vi "Find Exchanges.vi"(8 "error in (no error)":errorcluster caption="entrée d'erreur (pas d'erreur)", 10 "Position":i32, 11 "Exchanges en entrée":refnum<class "Exchanges.lvclass"> caption="DNL_LabVIEW Object in") -> (0 "error out":errorcluster caption="sortie d'erreur", 1 "Parameters":T1, 2 "found?":bool, 3 "Exchanges en sortie":refnum<class "Exchanges.lvclass"> caption="DNL_LabVIEW Object out")   [LabVIEW 2012, in "Exchanges.lvclass"]
uses:
  Exchanges.lvclass
  Exchange/Exchange Parameters.ctl
  Exchange/Exchange Type Enum.ctl
  controls/Currencies.ctl
  Exchanges.lvclass/Exchanges.ctl
  Exchange/Exchange.lvclass
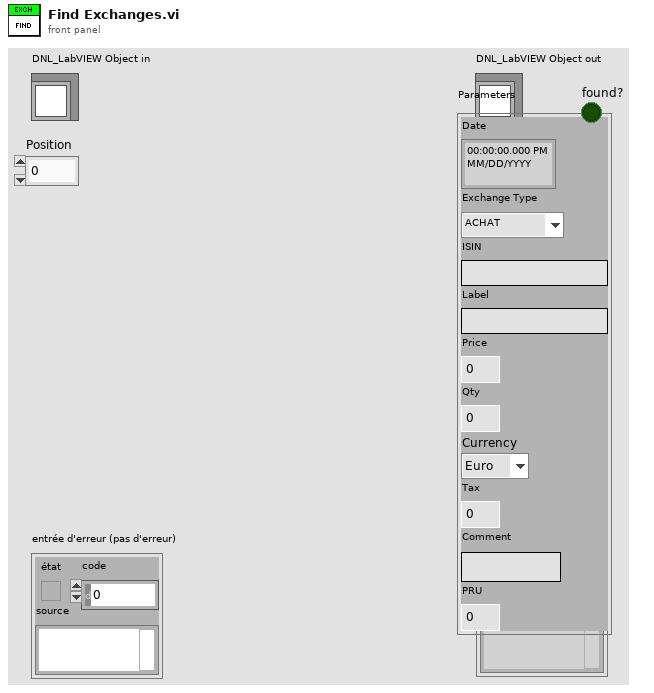
[diagram p1: front panel]
types:
  T1 = typedef "Exchange Parameters.ctl" = cluster{"Date":timestamp, "Exchange Type":T2, "ISIN":string, "Label":string, "Price":dbl, "Qty":dbl, "Currency":T3, "Tax":dbl, "Comment":string, "PRU":dbl}
  T2 = typedef "Exchange.lvclass/Exchange Type Enum.ctl" = enum16{"ACHAT", "VENTE"}
  T3 = typedef "Currencies.ctl" = enum16{"Euro", "Dollar", "Yen", "RIM", "CHF"}
  T4 = typedef "Dictionary Object RefNum__ogtk.ctl" = refnum<k1>
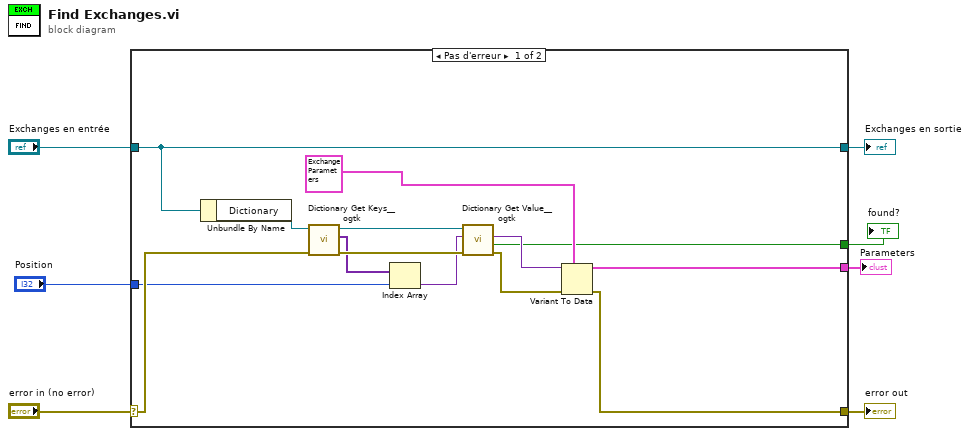
[diagram p0: block diagram]
diagram:
  n1 = case shown="Pas d'erreur" "error in (no error)" {
    selector: "error in (no error)" -> [w14 w23]
    tunnel: [w13 w23] -> w6
    tunnel: [w12 w22] -> w4
    tunnel: "Exchanges en entrée" -> [w12 w22]
    tunnel: [w10 _] -> w3
    tunnel: [w9 _] -> w2
    tunnel: "Position" -> [w8 _]
    frame No Error {
      n2 = Unbundle By Name(w12) -> ("Dictionary"=w18:T4)
      n3 = call <userlib>:"Dictionary Get Keys__ogtk.vi"("error in (no error)"=w14, "dictionary"=w18) -> ("error out"=w19:errorcluster, "keys"=w16:variant[], "dictionary out"=w17:T4)  [unwired: 7 in]
      n4 = Index Array(array=w16, index=w8) -> (element=w15:variant)
      n5 = call <userlib>:"Dictionary Get Value__ogtk.vi"("error in"=w19, "key"=w15, "dictionary"=w17) -> ("error out"=w20:errorcluster, "found?"=w9:bool, "value"=w21:variant)  [unwired: 5 in, 1 out]
      n6 = Variant To Data(error in=w20, type=T1 {"Date"=timestamp(0 s since 1904-01-01), "Exchange Type"=enum."ACHAT", "ISIN"="", "Label"="", "Price"=0.0, "Qty"=0.0, "Currency"=enum."Euro", "Tax"=0.0, "Comment"="", "PRU"=0.0} ("Parameters"), Variant=w21) -> (data=w10:T1, error out=w13:errorcluster)
    }
    frame Error {
    }
  }
  "error out" <- w6
  "Exchanges en sortie" <- w4
  "Parameters" <- w3
  "found?" <- w2
